vi "Load to memory.vi"(0 "Py Doc in":refnum<class "Py Doc.lvclass">, 5 "Path":path, 11 "error in (no error)":errorcluster) -> (4 "Py Doc out":refnum<class "Py Doc.lvclass">, 15 "error out":errorcluster)   [LabVIEW 2016, in "Py Doc.lvclass"]
uses:
  Py Doc.lvclass
  D:/MDI Project/source code/Document/Document.lvclass
  <vilib>/Utility/sysdir.llb/System Directory Type.ctl
  Document.lvclass/Document.ctl
  user32.dll
  Document.lvclass
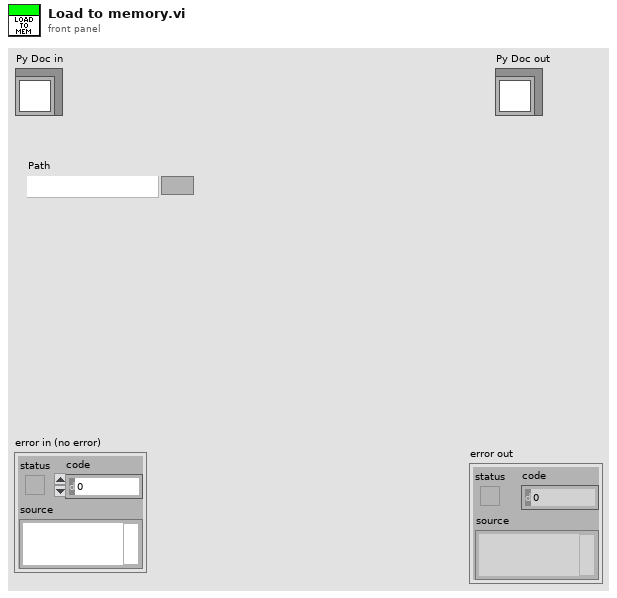
[diagram p1: front panel]
types:
  T1 = typedef "System Directory Type.ctl" = i32
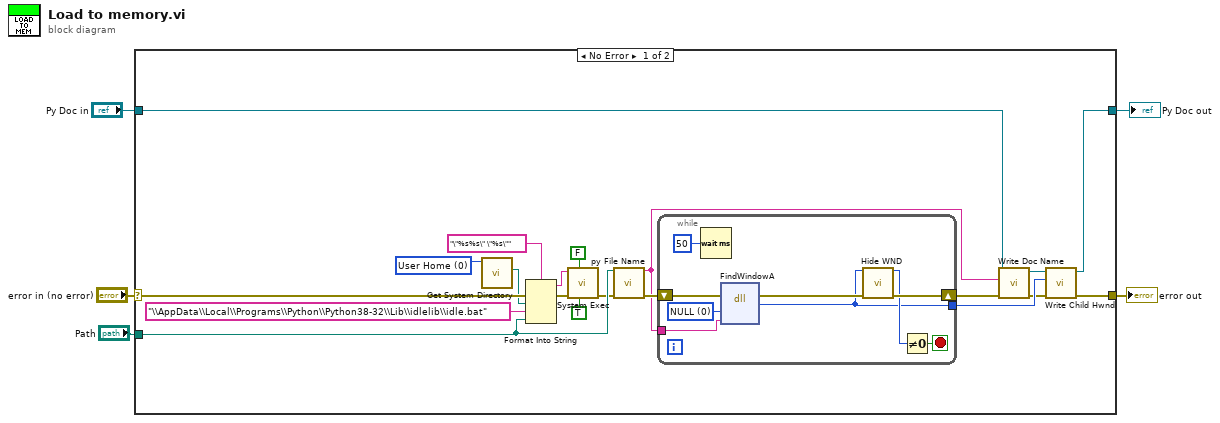
[diagram p0: block diagram]
diagram:
  n1 = case shown="No Error" "error in (no error)" {
    selector: "error in (no error)" -> [w25 w36]
    tunnel: [w6 w36] -> w4
    tunnel: "Py Doc in" -> [w10 w35]
    tunnel: [w9 w35] -> w2
    tunnel: "Path" -> [w17 _]
    frame No Error {
      w18 = T1 0 items=["User Home"=0, "User Desktop"=1, "User Documents"=2, "User Application Data"=3, "User Preferences"=4, "User Temporary"=5, "Public Documents"=6, "Public Application Data"=7, "Public Preferences"=8, "Public Cache"=13, "System Core Libraries"=9, "System Installed Libraries"=10, "Application Files"=11, "Boot Volume Root"=12] ("system directory type")
      n2 = call <vilib>:"Get System Directory.vi"("system directory type"=w18) -> ("system directory"=w15:path)  [unwired: 10 in]
      n3 = Format Into String(format string="\"%s%s\" \"%s\"", error in=w25, w15, "\\AppData\\Local\\Programs\\Python\\Python38-32\\Lib\\idlelib\\idle.bat" ("input 2"), w17) -> (resulting string=w23:string, error out=w24:errorcluster)  [unwired: 1 in]
      n4 = call <vilib>:"System Exec.vi"("run minimized? (F)"=TRUE, "wait until completion? (T)"=FALSE, "error in (no error)"=w24, "command line"=w23) -> ("error out"=w14:errorcluster)  [unwired: 4 in, 3 out]
      n5 = call "py File Name.vi"("Path"=w17, "error in (no error)"=w14) -> ("String"=w13:string, "error out"=w20:errorcluster)  [unwired: 12 in]
      n6 = while {
        tunnel: w13 -> [w30]
        tunnel: [w27] -> w12
        shift-right: [w32] -> w7
        shift-left: w20 -> [w31]
        stop <- w28 stop-if-true
        w34 = 0 items=["NULL"]
        n7 = Wait (ms)(milliseconds to wait=u32 50) -> ()  [unwired: 1 out]
        n8 = dll-call lib="user32.dll" fn="FindWindowA"(error in=w31, "lpzsClassName"=w34, "lpzsWindowName"=w30) -> (error out=w33:errorcluster, "hwnd"=w27:u32)  [unwired: 4 in, 1 out]
        n9 = call "Hide WND.vi"("hwnd"=w27, "error in (no error)"=w33) -> ("bool"=w29:u32, "error out"=w32:errorcluster)  [unwired: 12 in]
        n10 = Not Equal To 0?(x=w29) -> (x != 0?=w28:bool)
      }
      n11 = call "Write Doc Name.vi"("error in (no error)"=w7, "Doc Name"=w13, "Document in"=w10) -> ("error out"=w8:errorcluster, "Document out"=w11:refnum<class "Py Doc.lvclass">)  [unwired: 7 in]
      n12 = call "Write Child Hwnd.vi"("error in (no error)"=w8, "Child Hwnd"=w12, "Document in"=w11) -> ("error out"=w6:errorcluster, "Document out"=w9:refnum<class "Py Doc.lvclass">)  [unwired: 7 in]
    }
    frame Error {
    }
  }
  "error out" <- w4
  "Py Doc out" <- w2
